vi "Get Macro.vi"   [LabVIEW 2016, in "Hardware.lvlib" / "Motions.lvlib" / "Motions.lvclass"]
uses:
  <userlib>/Common Components/Hardware/Abstract System/Motions/Motions/Motions.lvclass
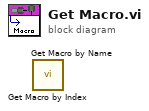
[diagram p0: block diagram]
diagram:
  n1 = call <userlib>:"Get Macro by Index.vi"() -> ()  [unwired: 8 in, 4 out]
  n2 = call <userlib>:"Get Macro by Name.vi"() -> ()  [unwired: 8 in, 4 out]
